vi "createPubDataEvents.vi"(8 "error in (no error)":errorcluster, 11 "UserEvents in":refnum<class "UserEvents.lvclass">) -> (0 "error out":errorcluster, 3 "UserEvents out":refnum<class "UserEvents.lvclass">)   [LabVIEW 2013, in "UserEvents.lvclass"]
uses:
  UserEvents.lvclass
  Typedefs/StateSelector.ctl
  Typedefs/InputData.ctl
  <userlib>/Common/ILC/Typedefs/ADCs.ctl
  Typedefs/OutputData.ctl
  Typedefs/TestStatus.ctl
  Typedefs/TemperatureSettling.ctl
  Typedefs/WaitTimeStatus.ctl
  UserEvents.lvclass/UserEvents.ctl
  Typedefs/AITDTTypedefs.lvlib
  <userlib>/Common/ILC/Typedefs/ILCTypedefs.lvlib
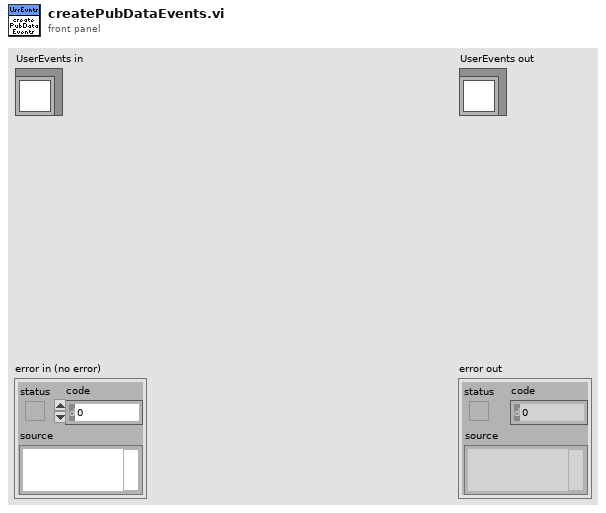
[diagram p1: front panel]
types:
  T1 = typedef "AITDTTypedefs.lvlib/WaitTimeStatus.ctl" = cluster{"Time Remaining":dbl[unit]}
  T2 = typedef "AITDTTypedefs.lvlib/TemperatureSettling.ctl" = cluster{"Temperature Measured":dbl[unit], "TemperatureSettledIsTrue":bool, "Required":cluster{"Sample Size Rqd":u16, "StDev":dbl[unit]}, "Measured":cluster{"StDev Msd":dbl[unit], "Sample Size Msd":u16}}
  T3 = typedef "AITDTTypedefs.lvlib/TestStatus.ctl" = cluster{"activeCycle":u32, "activeProfileStep":u32, "demandedCycles":u32, "demandedProfileSteps":u32, "temperatureSetpoint":dbl[unit], "pgaGainCoefficient":u16}
  T4 = typedef "AITDTTypedefs.lvlib/OutputData.ctl" = cluster{"Step & Direction":i16}
  T5 = typedef "AITDTTypedefs.lvlib/InputData.ctl" = cluster{"Temperature Measured":dbl[unit], "ADCs":T6}
  T6 = typedef "ILCCommon.lvlib/ILCTypedefs.lvlib/ADCs.ctl" = cluster{"Ch0":i32, "Ch1":i32, "Ch2":i32, "Ch3":i32, "Ch4":i32}
  T7 = typedef "AITDTTypedefs.lvlib/StateSelector.ctl" = enum16{"AwaitingSetpointAcknowledgmentState", "EndingCycleState", "FaultState", "OffState", "PausingState", "RequestingNewSetpointState", "SamplingState", "SettlingState", "SoakingState", "StabilizingState", "StandbyState", "StoppedState", "TransitioningTemperatureState"}
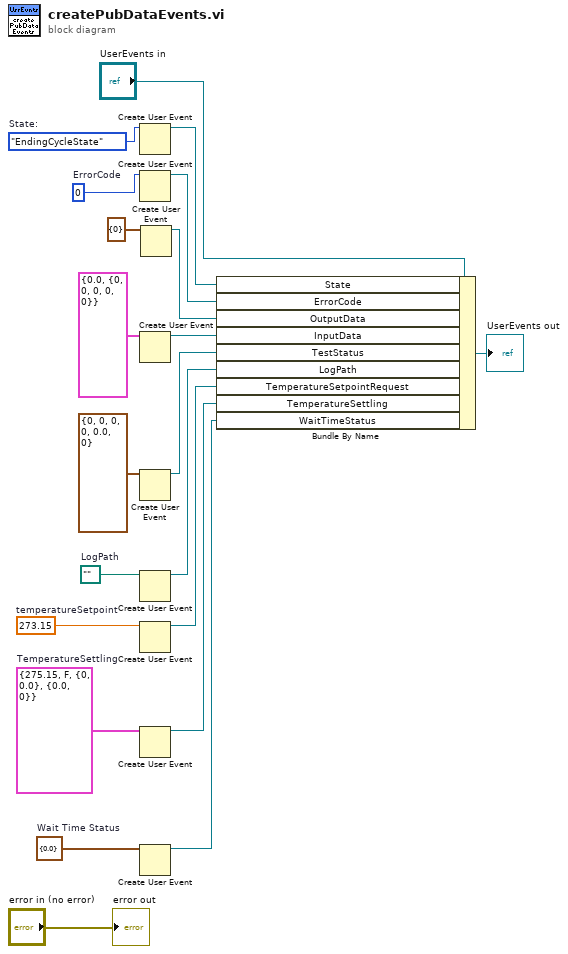
[diagram p0: block diagram]
diagram:
  w2 = T1 {"Time Remaining"=0.0}  # Wait Time Status
  w4 = T2 {"Temperature Measured"=275.15, "TemperatureSettledIsTrue"=FALSE, "Required"={"Sample Size Rqd"=0, "StDev"=0.0}, "Measured"={"StDev Msd"=0.0, "Sample Size Msd"=0}}  # TemperatureSettling
  w6 = dbl[unit] 273.15  # temperatureSetpoint
  w8 = path ""  # LogPath
  w17 = 0  # ErrorCode
  w18 = StateSelector."EndingCycleState"  # State:
  n1 = Create User Event(user event datatype=w18) -> (user event=w16:refnum<user-event>)  [unwired: 1 in, 1 out]
  n2 = Create User Event(user event datatype=w17) -> (user event=w15:refnum<user-event>)  [unwired: 1 in, 1 out]
  n3 = Create User Event(user event datatype=T5 {"Temperature Measured"=0.0, "ADCs"={"Ch0"=0, "Ch1"=0, "Ch2"=0, "Ch3"=0, "Ch4"=0}} ("Input Data")) -> (user event=w13:refnum<user-event>)  [unwired: 1 in, 1 out]
  n4 = Create User Event(user event datatype=T3 {"activeCycle"=0, "activeProfileStep"=0, "demandedCycles"=0, "demandedProfileSteps"=0, "temperatureSetpoint"=0.0, "pgaGainCoefficient"=0} ("TestStatus")) -> (user event=w9:refnum<user-event>)  [unwired: 1 in, 1 out]
  n5 = Create User Event(user event datatype=w8) -> (user event=w7:refnum<user-event>)  [unwired: 1 in, 1 out]
  n6 = Create User Event(user event datatype=w6) -> (user event=w5:refnum<user-event>)  [unwired: 1 in, 1 out]
  n7 = Create User Event(user event datatype=w4) -> (user event=w3:refnum<user-event>)  [unwired: 1 in, 1 out]
  n8 = Create User Event(user event datatype=w2) -> (user event=w1:refnum<user-event>)  [unwired: 1 in, 1 out]
  n9 = Create User Event(user event datatype=T4 {"Step & Direction"=0} ("Output Data")) -> (user event=w11:refnum<user-event>)  [unwired: 1 in, 1 out]
  n10 = Bundle By Name(cluster="UserEvents in", "State"=w16, "ErrorCode"=w15, "OutputData"=w11, "InputData"=w13, "TestStatus"=w9, "LogPath"=w7, "TemperatureSetpointRequest"=w5, "TemperatureSettling"=w3, "WaitTimeStatus"=w1) -> (→"UserEvents out":refnum<class "UserEvents.lvclass">)
  "error out" <- "error in (no error)"
